vi "Find Port.vi"(8 "error in":errorcluster, 10 "port number":u32, 11 "Ballard ARINC 429 custom device in":T1 format="%.0x") -> (0 "error out":errorcluster, 2 "port":T1 format="%.0x", 3 "Ballard ARINC 429 custom device out":T1 format="%.0x", 4 "found?":bool)   [LabVIEW 2020, in "AIM ARINC 429 Scripting.lvlib"]
doc: "Within the specified <b>Ballard ARINC 429 custom device in</b>, searches for an instance of <b>port</b> with matching hardware channel number. If a match is found, returns the matching <b>port</b> reference. If no match is found, the returned reference is invalid and <b>found?</b> equals False."
uses:
  AIM ARINC 429 Scripting.lvlib
  <vilib>/NI VeriStand/Custom Device API/Custom Device Item Ref.ctl
  ARINC 429/ARINC 429 Scripting.lvlib
  <vilib>/NI VeriStand/Custom Device API/Custom Device API.lvlib
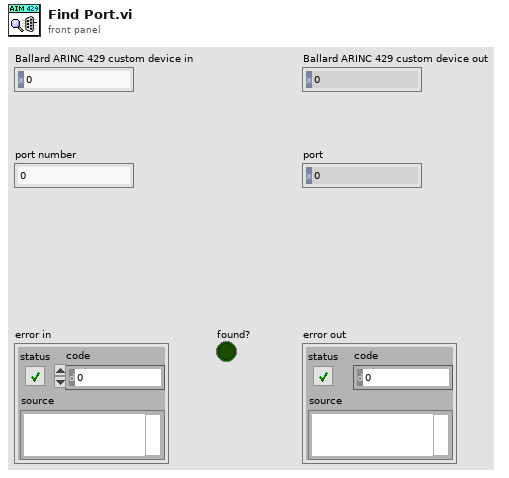
[diagram p1: front panel]
types:
  T1 = typedef "Custom Device API.lvlib/Custom Device Item Ref.ctl" = u64
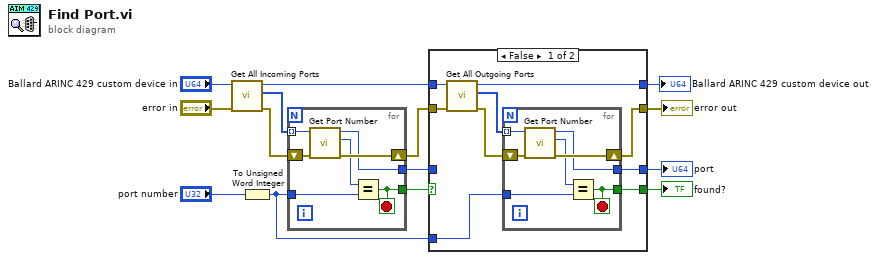
[diagram p0: block diagram]
diagram:
  n1 = call "Get All Incoming Ports.vi"("error in"="error in", "Ballard ARINC 429 custom device in"="Ballard ARINC 429 custom device in") -> ("error out"=w8:errorcluster, "incoming ports"=w9:T1[], "Ballard ARINC 429 custom device out"=w13:T1)  [unwired: 7 in]
  n2 = To Unsigned Word Integer(number="port number") -> (unsigned 16bit integer=w1:u16)
  n3 = for {
    tunnel: w9 -> [w21] mode=indexing
    shift-right: [w19] -> w5
    shift-left: w8 -> [w20]
    tunnel: w1 -> [w18]
    tunnel: [w17] -> w6
    tunnel: [w15] -> w4
    stop <- w17 stop-if-true
    n4 = call "Get Port Number.vi"("error in"=w20, "port ref in"=w21) -> ("error out"=w19:errorcluster, "port number"=w16:u16, "port ref out"=w15:T1)  [unwired: 6 in, 1 out]
    n5 = Equal?(x=w16, y=w18) -> (x = y?=w17:bool)
  }
  n6 = case shown="False" w6 {
    selector: w6 -> [_ w38]
    tunnel: w13 -> [w30 w41]
    tunnel: [w29 w41] -> w12
    tunnel: [w22 w40] -> w10
    tunnel: w5 -> [w28 w40]
    tunnel: w4 -> [_ w39]
    tunnel: [w27 w39] -> w3
    tunnel: [w23 w38] -> w2
    tunnel: w1 -> [w24 _]
    frame False {
      n7 = call "Get All Outgoing Ports.vi"("error in"=w28, "Ballard ARINC 429 custom device in"=w30) -> ("error out"=w26:errorcluster, "outgoing ports"=w25:T1[], "Ballard ARINC 429 custom device out"=w29:T1)  [unwired: 7 in]
      n8 = for {
        tunnel: w25 -> [w37] mode=indexing
        shift-right: [w35] -> w22
        shift-left: w26 -> [w36]
        tunnel: w24 -> [w34]
        tunnel: [w33] -> w23
        tunnel: [w31] -> w27
        stop <- w33 stop-if-true
        n9 = call "Get Port Number.vi"("error in"=w36, "port ref in"=w37) -> ("error out"=w35:errorcluster, "port number"=w32:u16, "port ref out"=w31:T1)  [unwired: 6 in, 1 out]
        n10 = Equal?(x=w32, y=w34) -> (x = y?=w33:bool)
      }
    }
    frame True {
    }
  }
  "port" <- w3
  "error out" <- w10
  "Ballard ARINC 429 custom device out" <- w12
  "found?" <- w2
